vi "Indicator Init.vi"(7 "VolatusAPI":refnum<class "VolatusAPI.lvclass">, 8 "error in (no error)":errorcluster, 10 "JSON":string, 11 "DblNumericStatusIndicator in":refnum<class "DblStatusIndicator.lvclass">) -> (0 "error out":errorcluster, 3 "DblNumericStatusIndicator out":refnum<class "DblStatusIndicator.lvclass">)   [LabVIEW 2020, in "VolatusGUIElements.lvlib" / "DblStatusIndicator.lvclass"]
uses:
  DblStatusIndicator.lvclass
  C:/dev/lv20CE/relink/lv-volatus/VolatusGUI/GUI Element/GUI Element.lvclass
  Volatus/VolatusAPI/VolatusAPI.lvclass
  JSON.ctl
  lv-vecto/Vecto/Group/Group.lvclass
  C:/dev/lv20CE/relink/lv-vecto/Vecto/GroupAbstract/GroupAbstract.lvclass
  VolatusGUI/GUI Element/GUI Element.lvclass/GUI Element.ctl
  DblStatusIndicator.lvclass/DblStatusIndicator.ctl
  c840d708-a4aa-4e42-9474-a77b72826cb9.vi
  <vilib>/JDP Science/JSONtext/JSON text to Variant.vi
  <vilib>/JDP Science/JSONtext/LVClass Serializer/JSONtext LVClass Serializer.lvclass
  VolatusGUI/GUI Element/GUI Element.lvclass
  VolatusGUIElements.lvlib
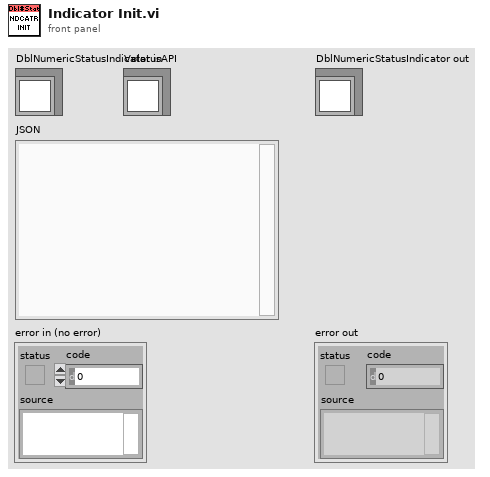
[diagram p1: front panel]
types:
  T1 = typedef "VolatusGUIElements.lvlib/DblStatusIndicator.lvclass/JSON.ctl" = cluster{"Group":string, "Channel":string, "Staleness":dbl, "Format":string, "Color":string}
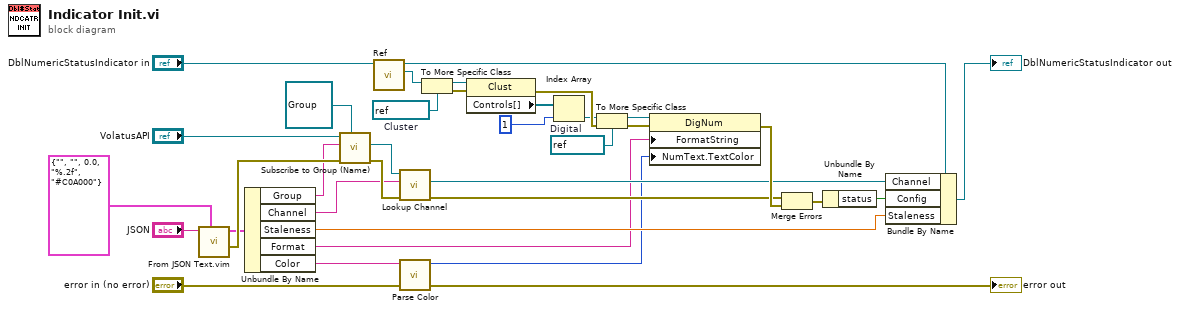
[diagram p0: block diagram]
diagram:
  w8 = refnum<vi> refnum  # Digital
  w13 = refnum<vi> refnum  # Cluster
  n1 = call "From JSON Text.vim"("Data Type and Default Value"=T1 {"Group"="", "Channel"="", "Staleness"=0.0, "Format"="%.2f", "Color"="#C0A000"} ("JSON"), "JSON"="JSON") -> ("error out"=w32:errorcluster, "Data out"=w29:T1)  [unwired: 8 in]
  n2 = Unbundle By Name(w29) -> ("Group"=w23:string, "Channel"=w22:string, "Staleness"=w21:dbl, "Format"=w4:string, "Color"=w2:string)
  n3 = call "Subscribe to Group (Name).vi"("Group Type"=refnum<class "Group.lvclass"> refnum ("Group in"), "error in (no error)"=w32, "Group Name"=w23, "VolatusAPI in"="VolatusAPI") -> ("error out"=w28:errorcluster, "Group"=w25:refnum<class "Group.lvclass">)  [unwired: 5 in, 1 out]
  n4 = call "Ref.vi"("GUI Element in"="DblNumericStatusIndicator in") -> ("Ref"=w14:refnum<vi>, "GUI Element out"=w16:refnum<class "DblStatusIndicator.lvclass">)  [unwired: 9 in]
  n5 = call "Lookup Channel.vi"("error in (no error)"=w28, "Channel Name"=w22, "Group in"=w25) -> ("error out"=w12:errorcluster, "Channel"=w27:refnum<class "Channel.lvclass">)  [unwired: 6 in, 1 out]
  n6 = call "Parse Color.vi"("Color String"=w2) -> ("Color"=w1:u32)  [unwired: 9 in, 1 out]
  n7 = To More Specific Class(target class=w13, reference=w14) -> (specific class reference=w15:refnum<vi>, error out=w5:errorcluster)  [unwired: 1 in]
  n8 = property class="Clust"(reference=w15, error in=w5) -> (error out=w33:errorcluster, "Controls[]"=w10:refnum<vi>[])  [unwired: 1 out]
  n9 = Index Array(array=w10, index=1) -> (element=w9:refnum<vi>)
  n10 = To More Specific Class(target class=w8, reference=w9, error in=w33) -> (specific class reference=w7:refnum<vi>, error out=w6:errorcluster)
  n11 = property class="DigNum"(reference=w7, error in=w6, "FormatString"=w4, "NumText.TextColor"=w1) -> (error out=w34:errorcluster)  [unwired: 1 out]
  n12 = Merge Errors(w12, w34) -> (w11:errorcluster)
  n13 = Unbundle By Name(w11) -> ("status"=w18:bool)
  n14 = Bundle By Name(cluster=w16, "Channel"=w27, "Config"=w18, "Staleness"=w21) -> (→"DblNumericStatusIndicator out":refnum<class "DblStatusIndicator.lvclass">)
  "error out" <- "error in (no error)"
